vi "Autoengager.vi"(0 "Main Interface":T1, 1 "Focus and Tracking":T5, 2 "System of Reference Interface":T2, 3 "Guided Approach Calibration":T7, 4 "Approach Target Button":refnum<vi>, 5 "Target":T4, 9 "Tip":T3, 11 "Error In":errorcluster, 12 "Manipulator Interface":T8, 13 "Start Coordinates [pix]":refnum<vi>, 14 "Calibration":T6) -> (6 "Done":bool, 8 "Aborted":bool, 10 "Scope Error":bool, 15 "Error Out":errorcluster)   [LabVIEW 2012, in "Targeting Unit.lvlib"]
uses:
  Targeting Unit.lvlib
  <vilib>/Analysis/Matrix/Datatypes/RealMatrix.ctl
  <vilib>/Analysis/Matrix/NI_Matrix.lvlib
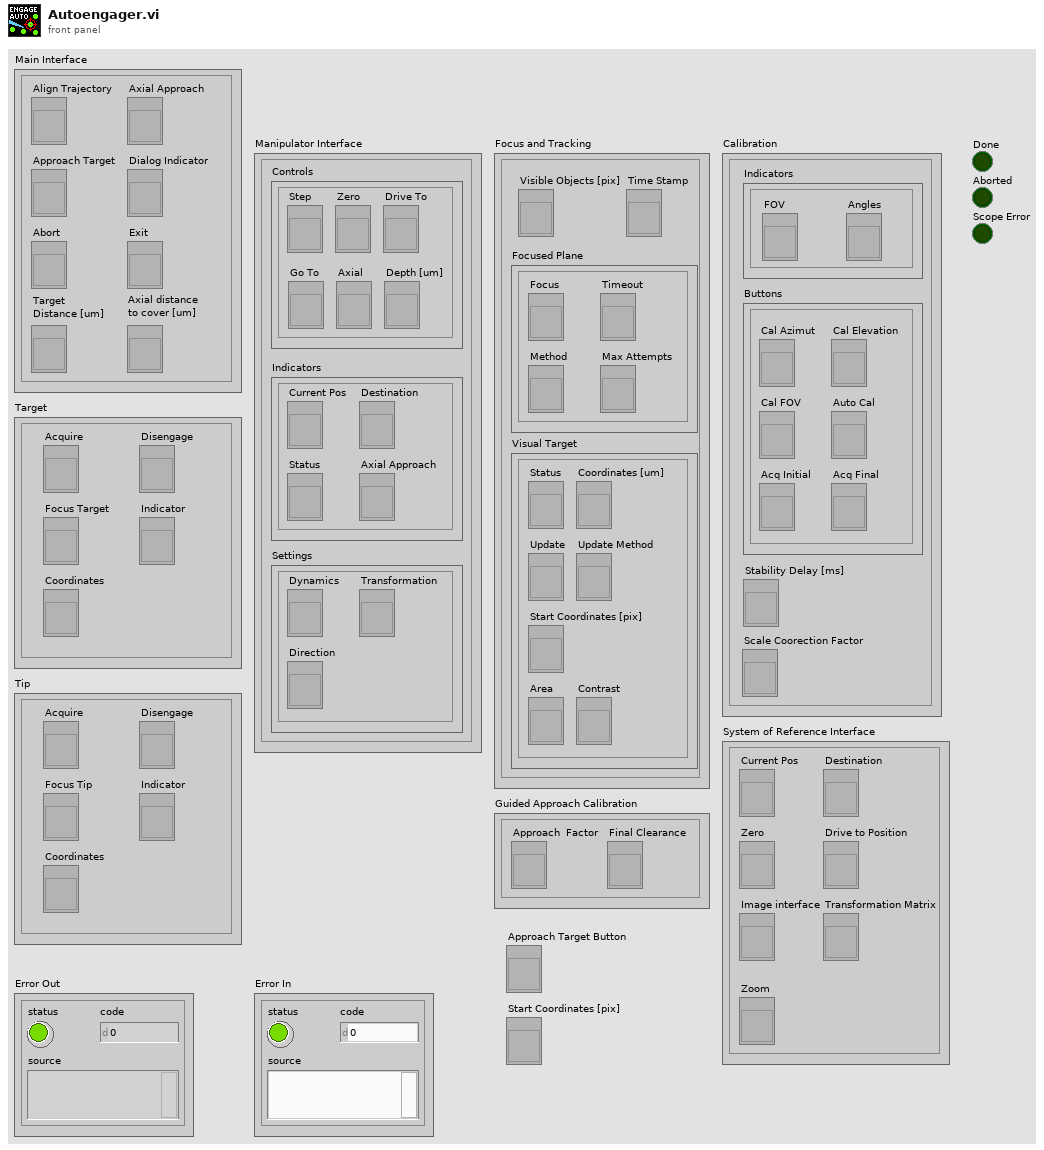
[diagram p1: front panel]
types:
  T1 = cluster{"Exit":refnum<vi>, "Abort":refnum<vi>, "Align Trajectory":refnum<vi>, "Axial Approach":refnum<vi>, "Dialog Indicator":refnum<vi>, "Approach Target":refnum<vi>, "Target\nDistance [um]":refnum<vi>, "Axial distance \nto cover [um]":refnum<vi>}
  T2 = cluster{"Current Pos":refnum<vi>, "Image interface":refnum<vi>, "Transformation Matrix":refnum<vi>, "Zero":refnum<vi>, "Destination":refnum<vi>, "Drive to Position":refnum<vi>, "Zoom":refnum<vi>}
  T3 = cluster{"Coordinates":refnum<vi>, "Acquire":refnum<vi>, "Disengage":refnum<vi>, "Indicator":refnum<vi>, "Focus Tip":refnum<vi>}
  T4 = cluster{"Coordinates":refnum<vi>, "Acquire":refnum<vi>, "Disengage":refnum<vi>, "Indicator":refnum<vi>, "Focus Target":refnum<vi>}
  T5 = cluster{"Focused Plane":cluster{"Focus":refnum<vi>, "Timeout":refnum<vi>, "Max Attempts":refnum<vi>, "Method":refnum<vi>}, "Time Stamp":refnum<vi>, "Visual Target":cluster{"Coordinates [um]":refnum<vi>, "Status":refnum<vi>, "Update":refnum<vi>, "Update Method":refnum<vi>, "Start Coordinates [pix]":refnum<vi>, "Area":refnum<vi>, "Contrast":refnum<vi>}, "Visible Objects [pix]":refnum<vi>}
  T6 = cluster{"Indicators":cluster{"FOV":refnum<vi>, "Angles":refnum<vi>}, "Buttons":cluster{"Cal FOV":refnum<vi>, "Cal Azimut":refnum<vi>, "Cal Elevation":refnum<vi>, "Auto Cal":refnum<vi>, "Acq Initial":refnum<vi>, "Acq Final":refnum<vi>}, "Stability Delay [ms]":refnum<vi>, "Scale Coorection Factor":refnum<vi>}
  T7 = cluster{"Approach  Factor":refnum<vi>, "Final Clearance":refnum<vi>}
  T8 = cluster{"Indicators":cluster{"Current Pos":refnum<vi>, "Destination":refnum<vi>, "Status":refnum<vi>, "Axial Approach":refnum<vi>}, "Settings":cluster{"Dynamics":refnum<vi>, "Transformation":refnum<vi>, "Direction":refnum<vi>}, "Controls":cluster{"Zero":refnum<vi>, "Step":refnum<vi>, "Drive To":refnum<vi>, "Go To":refnum<vi>, "Axial":refnum<vi>, "Depth [um]":refnum<vi>}}
  T9 = cluster{"X [um]":dbl, "Y [um]":dbl, "Z [um]":dbl}
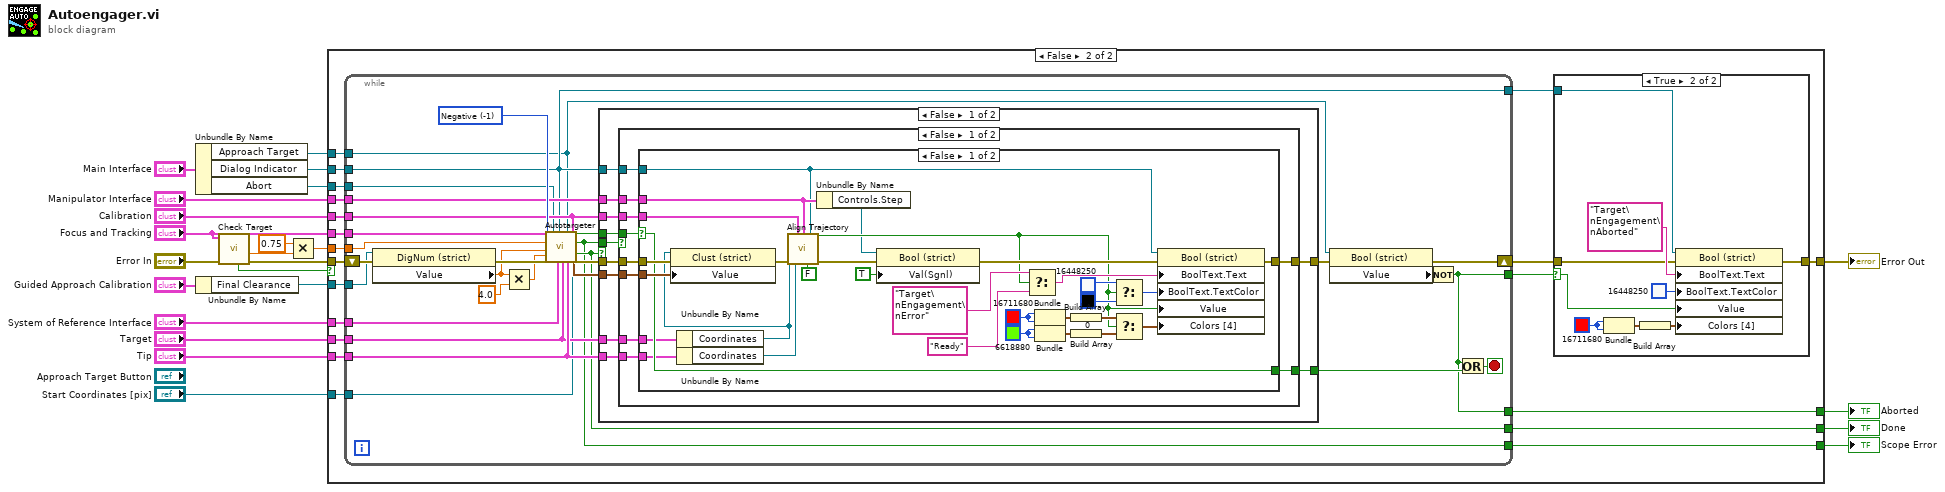
[diagram p0: block diagram]
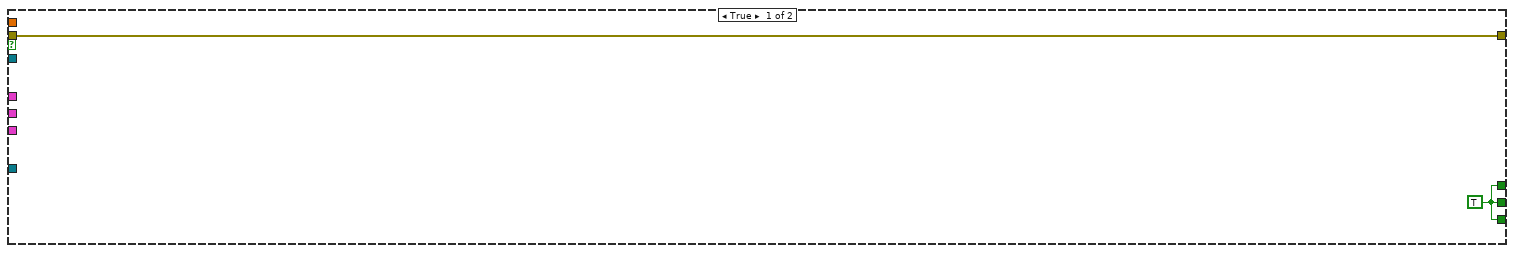
[diagram p2: hidden frame]
diagram:
  n1 = Unbundle By Name("Main Interface") -> ("Approach Target"=w16:refnum<vi>, "Dialog Indicator"=w15:refnum<vi>, "Abort"=w14:refnum<vi>)
  n2 = Unbundle By Name("Guided Approach Calibration") -> ("Final Clearance"=w12:refnum<vi>)
  n3 = call "Check Target.vi"("Error In"="Error In", "Focus and Tracking"="Focus and Tracking") -> ("Error out"=w5:errorcluster, "CFS"=w4:dbl, "Scope Error"=w1:bool)  [unwired: 3 in, 4 out]
  n4 = Multiply(x=0.75 ("y"), y=w4) -> (x*y=w2:dbl)
  n5 = case shown="False" w1 {
    tunnel: [w25 w42] -> w23
    tunnel: "Calibration" -> [_ w41]
    tunnel: "Manipulator Interface" -> [_ w40]
    tunnel: "Target" -> [_ w39]
    tunnel: "Tip" -> [_ w38]
    tunnel: "System of Reference Interface" -> [_ w37]
    tunnel: w16 -> [_ w36]
    tunnel: w15 -> [_ w35]
    tunnel: w14 -> [_ w34]
    tunnel: w12 -> [_ w33]
    tunnel: [w24 w32] -> w11
    tunnel: [w24 w31] -> w10
    tunnel: [w24 w30] -> w9
    tunnel: "Start Coordinates [pix]" -> [_ w29]
    tunnel: "Focus and Tracking" -> [_ w28]
    tunnel: w5 -> [w25 w27]
    tunnel: w2 -> [_ w26]
    frame True {
      w24 = TRUE
    }
    frame False {
      n6 = while {
        tunnel: [w48] -> w45
        tunnel: [w60] -> w43
        shift-right: [w69] -> w44
        shift-left: w27 -> [w57]
        tunnel: w35 -> [w60]
        tunnel: w41 -> [w66]
        tunnel: w28 -> [w65]
        tunnel: w40 -> [w64]
        tunnel: w39 -> [w61]
        tunnel: w38 -> [w62]
        tunnel: w37 -> [w63]
        tunnel: w34 -> [w59]
        tunnel: w36 -> [w58]
        tunnel: w33 -> [w52]
        tunnel: [w50] -> w32
        tunnel: [w49] -> w31
        tunnel: [w48] -> w30
        tunnel: w29 -> [w47]
        tunnel: w26 -> [w46]
        stop <- w67 stop-if-true
        w71 = i8 -1 items=["Positive"=1, "Negative"=-1] ("Z direction")
        n7 = property class="DigNum (strict)"(reference=w52, error in=w57) -> (error out=w56:errorcluster, "Value"=w54:dbl)  [unwired: 1 out]
        n8 = Multiply(x=w54, y=4.0) -> (x*y=w55:dbl)
        n9 = call "Autotargeter.vi"("Target"=w61, "Tip"=w62, "System of Reference Interface"=w63, "Refocus threshold"=w46, "Error In"=w56, "Focus and Tracking"=w65, "Maximal Clearance [um]"=w55, "Active"=w58, "Minimal Clearance [um]"=w54, "Dialog Indicator"=w60, "Z direction"=w71, "Calibration"=w66, "Abort"=w59, "Start Coordinates [pix]"=w47) -> ("Fail"=w73:bool, "Scope Error"=w49:bool, "Done"=w50:bool, "Target Coordinates"=w72:T9, "Error Out"=w74:errorcluster)  [unwired: 9 in]
        n10 = case shown="False" w50 {
          selector: w50 -> [_ w132]
          tunnel: [w84 w132] -> w51
          tunnel: w49 -> [w85 _]
          tunnel: w74 -> [w82 w131]
          tunnel: w73 -> [w83 _]
          tunnel: w60 -> [w81 _]
          tunnel: w72 -> [w80 _]
          tunnel: [w79 w131] -> w70
          tunnel: w66 -> [w78 _]
          tunnel: w64 -> [w77 _]
          tunnel: w62 -> [w76 _]
          tunnel: w61 -> [w75 _]
          frame False {
            n11 = case shown="False" w85 {
              selector: w85 -> [_ w130]
              tunnel: [w90 w130] -> w84
              tunnel: w83 -> [w95 _]
              tunnel: w82 -> [w93 w129]
              tunnel: w81 -> [w94 _]
              tunnel: w80 -> [w92 _]
              tunnel: [w91 w129] -> w79
              tunnel: w78 -> [w89 _]
              tunnel: w77 -> [w88 _]
              tunnel: w76 -> [w87 _]
              tunnel: w75 -> [w86 _]
              frame False {
                n12 = case shown="False" w95 {
                  selector: w95 -> [w119 w127]
                  tunnel: [w108 w128] -> w91
                  tunnel: w94 -> [w97 _]
                  tunnel: w93 -> [w121 w128]
                  tunnel: w92 -> [w120 _]
                  tunnel: [w119 w127] -> w90
                  tunnel: w89 -> [w105 _]
                  tunnel: w88 -> [w99 _]
                  tunnel: w87 -> [w102 _]
                  tunnel: w86 -> [w101 _]
                  frame False {
                    w112 = u32 6618880
                    w115 = u32 16711680
                    n13 = Unbundle By Name(w101) -> ("Coordinates"=w103:refnum<vi>)
                    n14 = property class="Clust (strict)"(reference=w103, error in=w121, "Value"=w120) -> (error out=w122:errorcluster)  [unwired: 1 out]
                    n15 = Unbundle By Name(w102) -> ("Coordinates"=w104:refnum<vi>)
                    n16 = call "Align Trajectory.vi"("Force alignemnt"=FALSE, "Indicator"=w97, "Calibration"=w105, "error in"=w122, "Tip Coordinates"=w104, "Target Coordinates"=w103, "Manipulator Interface"=w99) -> ("error out"=w123:errorcluster, "Error"=w100:bool)  [unwired: 3 in]
                    n17 = Unbundle By Name(w99) -> ("Controls.Step"=w98:refnum<vi>)
                    n18 = property class="Bool (strict)"(reference=w98, error in=w123, "Val(Sgnl)"=TRUE ("Value (Signaling)")) -> (error out=w107:errorcluster)  [unwired: 1 out]
                    n19 = Select(t="Target\nEngagement\nError", s=w100, f="Ready" ("t")) -> (s? t:f=w106:string)
                    n20 = Bundle(w115, w115) -> (w114:cluster{u32, u32})  [unwired: 1 in]
                    n21 = Bundle(w112, w112) -> (w111:cluster{u32, u32})  [unwired: 1 in]
                    n22 = Build Array(w114) -> (w113:cluster{u32, u32}[])
                    n23 = Build Array(w111) -> (w110:cluster{u32, u32}[])
                    n24 = Select(t=u32 16448250, s=w100, f=u32 0) -> (s? t:f=w116:u32)
                    n25 = Select(t=w113, s=w100, f=w110) -> (s? t:f=w109:cluster{u32, u32}[])
                    n26 = property class="Bool (strict)"(reference=w97, error in=w107, "BoolText.Text"=w106, "BoolText.TextColor"=w116, "Value"=w100, "Colors [4]"=w109) -> (error out=w108:errorcluster)  [unwired: 1 out]
                  }
                  frame True {
                    # "Fail"
                  }
                }
              }
              frame True {
                # "Scope Error"
              }
            }
          }
          frame True {
            # "Done"
          }
        }
        n27 = property class="Bool (strict)"(reference=w58, error in=w70) -> (error out=w69:errorcluster, "Value"=w68:bool)  [unwired: 1 out]
        n28 = Not(x=w68) -> (.not. x?=w48:bool)
        n29 = Or(x=w48, y=w51) -> (x .or. y?=w67:bool)
      }
      n30 = case shown="True" w45 {
        selector: w45 -> [_ w134]
        tunnel: w44 -> [w133 w137]
        tunnel: [w133 w136] -> w42
        tunnel: w43 -> [_ w135]
        frame False {
        }
        frame True {
          w139 = u32 16711680
          n31 = Bundle(w139, w139) -> (w138:cluster{u32, u32})  [unwired: 1 in]
          n32 = Build Array(w138) -> (w140:cluster{u32, u32}[])
          n33 = property class="Bool (strict)"(reference=w135, error in=w137, "BoolText.Text"="Target\nEngagement\nAborted" ("t"), "BoolText.TextColor"=u32 16448250, "Value"=w134, "Colors [4]"=w140) -> (error out=w136:errorcluster)  [unwired: 1 out]
        }
      }
    }
  }
  "Error Out" <- w23
  "Done" <- w11
  "Aborted" <- w9
  "Scope Error" <- w10
